vi "Mach_subvi.vi"(10 "Mach_IN":dbl, 11 "Mach_File":dbl[][](array[numeric])) -> (3 "OUT_Interp":dbl[](array[numeric]))   [LabVIEW 2017]
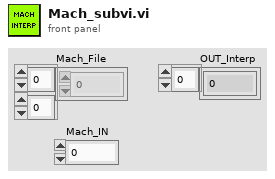
[diagram p1: front panel]
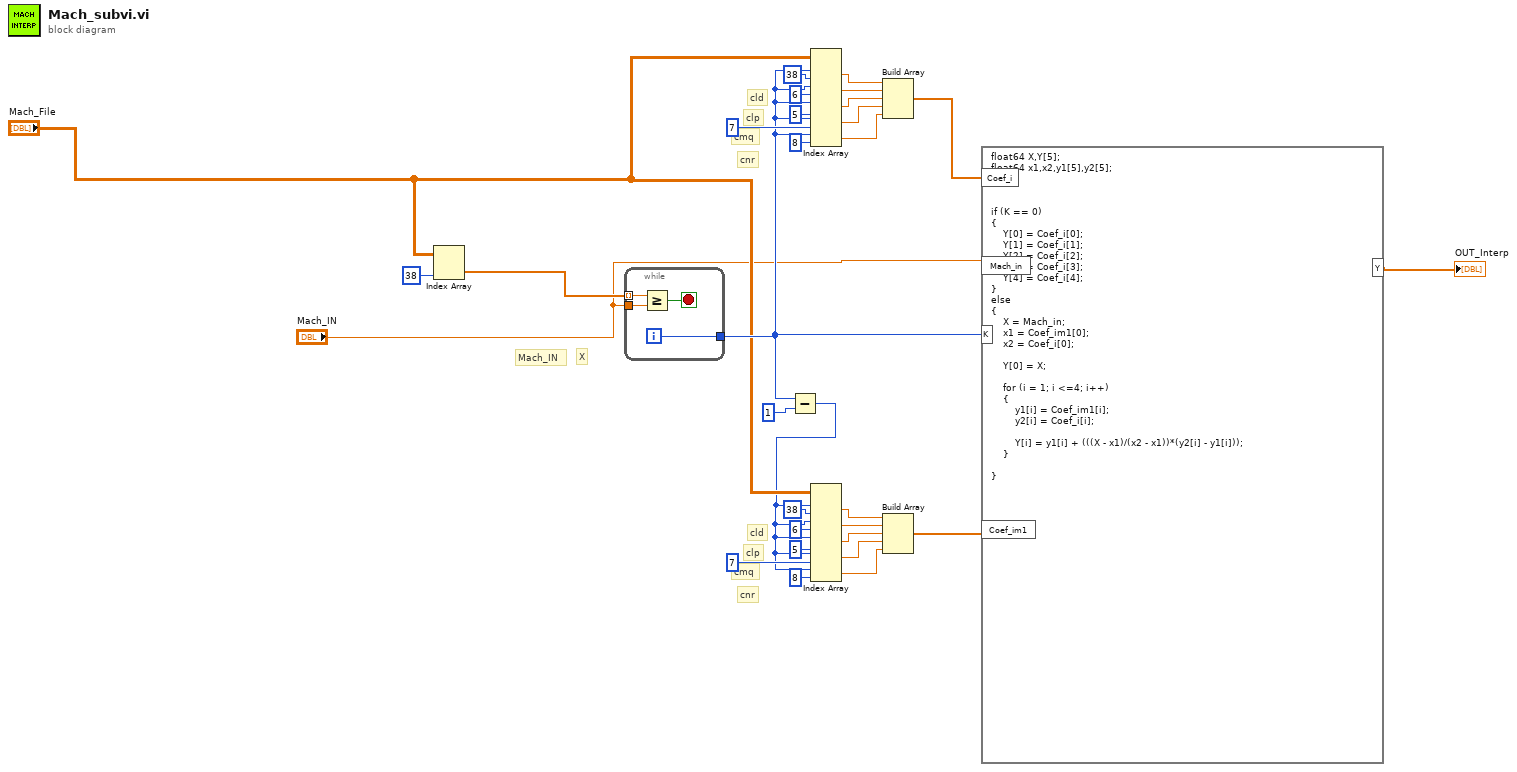
[diagram p0: block diagram]
diagram:
  # "cnr"
  # "cmq"
  # "clp"
  # "cld"
  # "cnr"
  # "cmq"
  # "clp"
  # "cld"
  # "X"
  # "Mach_IN"
  n1 = Index Array(array="Mach_File", index (col)=38 ("disabled index (col)")) -> (element=w30:dbl[])  [unwired: 1 in]
  n2 = while {
    tunnel: w30 -> [w33] mode=indexing
    tunnel: "Mach_IN" -> [w31]
    tunnel: [w32] -> w17
    i -> [w32]
    stop <- w34 stop-if-true
    n3 = Greater Or Equal?(x=w33, y=w31) -> (x >= y?=w34:bool)
  }
  n4 = Subtract(x=w17, y=1) -> (x-y=w4:i32)
  n5 = Index Array(array="Mach_File", index (row) #1=w17, index (col) #1=38 ("disabled index (col)"), index (row) #2=w17, index (col) #2=6 ("disabled index (col)"), index (row) #3=w17, index (col) #3=5 ("disabled index (col)"), index (row) #4=w17, index (col) #4=7 ("disabled index (col)"), index (row) #5=w17, index (col) #5=8 ("disabled index (col)")) -> (element #1=w23:dbl, element #2=w22:dbl, element #3=w21:dbl, element #4=w20:dbl, element #5=w19:dbl)
  n6 = Index Array(array="Mach_File", index (row) #1=w4, index (col) #1=38 ("disabled index (col)"), index (row) #2=w4, index (col) #2=6 ("disabled index (col)"), index (row) #3=w4, index (col) #3=5 ("disabled index (col)"), index (row) #4=w4, index (col) #4=7 ("disabled index (col)"), index (row) #5=w4, index (col) #5=8 ("disabled index (col)")) -> (element #1=w10:dbl, element #2=w9:dbl, element #3=w8:dbl, element #4=w7:dbl, element #5=w6:dbl)
  n7 = Build Array(w23, w22, w21, w20, w19) -> (w18:dbl[])
  n8 = Build Array(w10, w9, w8, w7, w6) -> (w3:dbl[])
  n9 = formula code="float64 X,Y[5];\nfloat64 x1,x2,y1[5],y2[5];\nint i;\n\n\nif (K == 0)\n{\n    Y[0] = Coef_i[0];\n    Y[1] = Coef_i[1];\n    Y[2] = Coef_i[2];\n    Y[3] = Coef_i[3];\n    Y[4] = Coef_i[4];\n}\nelse\n{\n    X = Mach_in;\n    x1 = Coef_im1[0];\n    x2 = Coef_i[0];\n\n    Y[0] = X;\n\n    for (i = 1; i <=4; i++)\n    {\n        y1[i] = Coef_im1[i]; \n        y2[i] = Coef_i[i]; \n\n        Y[i] = y1[i] + (((X - x1)/(x2 - x1))*(y2[i] - y1[i])); \n    }\n\n}"("K"=w17, "Coef_i"=w18, "Coef_im1"=w3, "Mach_in"="Mach_IN") -> ("Y"=→"OUT_Interp":dbl[])
